vi "SGL to String.vi"(7 "enable LabVIEW extensions?":bool, 11 "SGL":sgl) -> (3 "SGL string":string)   [LabVIEW 2019, in "JSONtext.lvlib"]
uses:
  JSONtext.lvlib
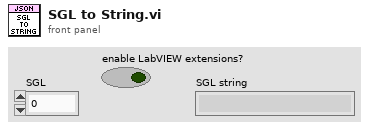
[diagram p1: front panel]
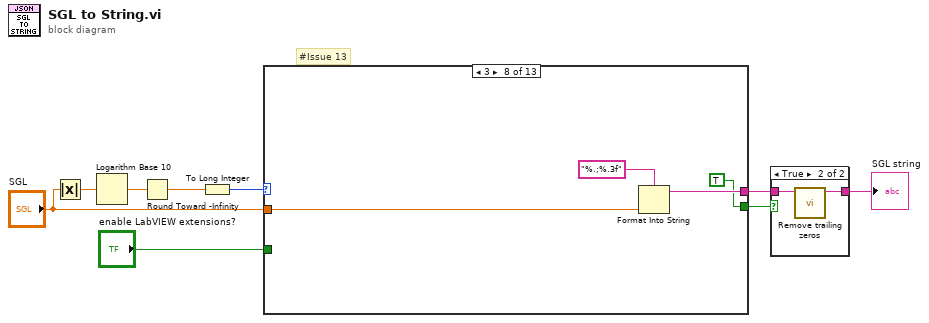
[diagram p0: block diagram]
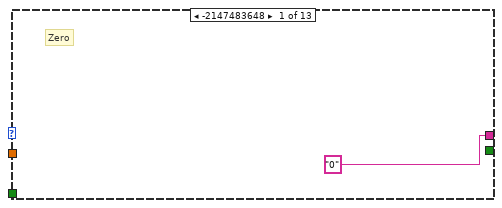
[diagram p3: hidden frame]
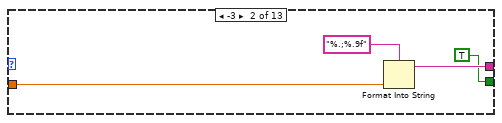
[diagram p4: hidden frame]
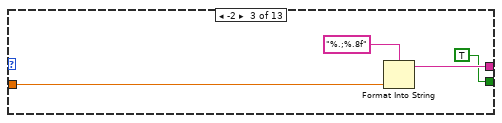
[diagram p5: hidden frame]
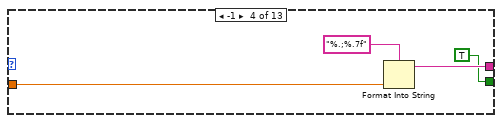
[diagram p6: hidden frame]
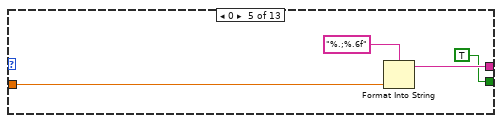
[diagram p7: hidden frame]
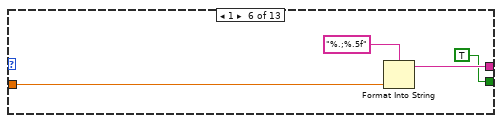
[diagram p8: hidden frame]
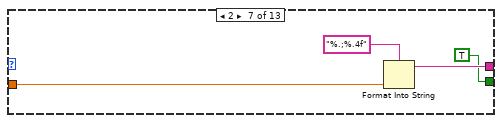
[diagram p9: hidden frame]
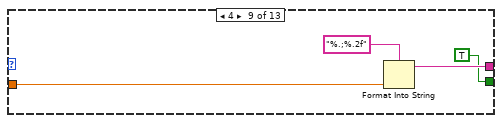
[diagram p10: hidden frame]
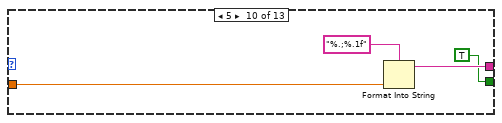
[diagram p11: hidden frame]
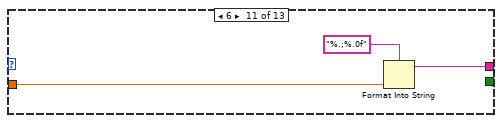
[diagram p12: hidden frame]
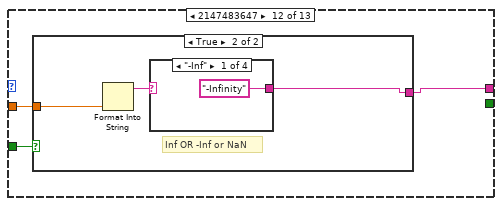
[diagram p13: hidden frame]
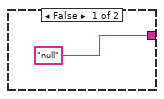
[diagram p14: hidden frame]
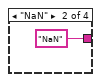
[diagram p15: hidden frame]
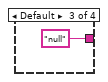
[diagram p16: hidden frame]
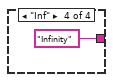
[diagram p17: hidden frame]
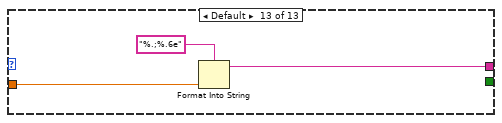
[diagram p18: hidden frame]
diagram:
  # "#Issue 13"
  n1 = Absolute Value(x="SGL") -> (abs(x)=w6:sgl)
  n2 = Logarithm Base 10(1:w6) -> (0:w3:sgl)
  n3 = Round Toward -Infinity(1:w3) -> (0:w4:sgl)
  n4 = To Long Integer(number=w4) -> (32bit integer=w5:i32)
  n5 = case shown="3" w5 {
    tunnel: ["0" w14 w18 w22 w26 w30 w34 w38 w42 w46 w49 w50 w62] -> w8
    tunnel: "SGL" -> [_ w13 w17 w21 w25 w29 w33 w37 w41 w45 w48 w52 w63]
    tunnel: "enable LabVIEW extensions?" -> [_ _ _ _ _ _ _ _ _ _ _ w51 _]
    tunnel: [_ TRUE TRUE TRUE TRUE TRUE TRUE TRUE TRUE TRUE _ _ _] -> w9
    frame -2147483648 {
      # "Zero"
    }
    frame -3 {
      n6 = Format Into String(format string="%.;%.9f", w13) -> (resulting string=w14:string)  [unwired: 2 in, 1 out]
    }
    frame -2 {
      n7 = Format Into String(format string="%.;%.8f", w17) -> (resulting string=w18:string)  [unwired: 2 in, 1 out]
    }
    frame -1 {
      n8 = Format Into String(format string="%.;%.7f", w21) -> (resulting string=w22:string)  [unwired: 2 in, 1 out]
    }
    frame 0 {
      n9 = Format Into String(format string="%.;%.6f", w25) -> (resulting string=w26:string)  [unwired: 2 in, 1 out]
    }
    frame 1 {
      n10 = Format Into String(format string="%.;%.5f", w29) -> (resulting string=w30:string)  [unwired: 2 in, 1 out]
    }
    frame 2 {
      n11 = Format Into String(format string="%.;%.4f", w33) -> (resulting string=w34:string)  [unwired: 2 in, 1 out]
    }
    frame 3 {
      n12 = Format Into String(format string="%.;%.3f", w37) -> (resulting string=w38:string)  [unwired: 2 in, 1 out]
    }
    frame 4 {
      n13 = Format Into String(format string="%.;%.2f", w41) -> (resulting string=w42:string)  [unwired: 2 in, 1 out]
    }
    frame 5 {
      n14 = Format Into String(format string="%.;%.1f", w45) -> (resulting string=w46:string)  [unwired: 2 in, 1 out]
    }
    frame 6 {
      n15 = Format Into String(format string="%.;%.0f", w48) -> (resulting string=w49:string)  [unwired: 2 in, 1 out]
    }
    frame 2147483647 {
      n16 = case shown="True" w51 {
        tunnel: w52 -> [_ w55]
        tunnel: ["null" w54] -> w50
        frame False {
        }
        frame True {
          # "Inf OR -Inf or NaN"
          n17 = Format Into String(w55) -> (resulting string=w56:string)  [unwired: 3 in, 1 out]
          n18 = case shown="\"-Inf\"" w56 {
            tunnel: ["-Infinity" "NaN" "null" "Infinity"] -> w54
            frame "-Inf" {
            }
            frame "NaN" {
            }
            frame Default {
            }
            frame "Inf" {
            }
          }
        }
      }
    }
    frame Default {
      n19 = Format Into String(format string="%.;%.6e", w63) -> (resulting string=w62:string)  [unwired: 2 in, 1 out]
    }
  }
  n20 = case shown="True" w9 {
    tunnel: [w64 w66] -> w7
    tunnel: w8 -> [w64 w65]
    frame False {
    }
    frame True {
      n21 = call "Remove trailing zeros.vi"("Number"=w65) -> ("Number with trainlg zeros removed"=w66:string)  [unwired: 10 in]
    }
  }
  "SGL string" <- w7
